vi "color.vi"(8 "error in":errorcluster, 11 "Stop (F) in":bool caption="Stop (F)") -> (0 "error out":errorcluster, 1 "blue":i32, 2 "red":i32, 3 "Refnum out":T1(plugin-control), 4 "yellow":i32, 5 "green":i32, 6 "Matches (Color Location 1) 2":T2(array[cluster]) {"Bounding Box"."y" format="%.2f"; "Bounding Box"."x" format="%.2f"; "Position"."y" format="%.2f"; "Position"."x" format="%.2f"; "Score" format="%.2f"; "Scale" format="%.2f"; "Angle" format="%.2f"}, 7 "black":i32)   [LabVIEW 2019]
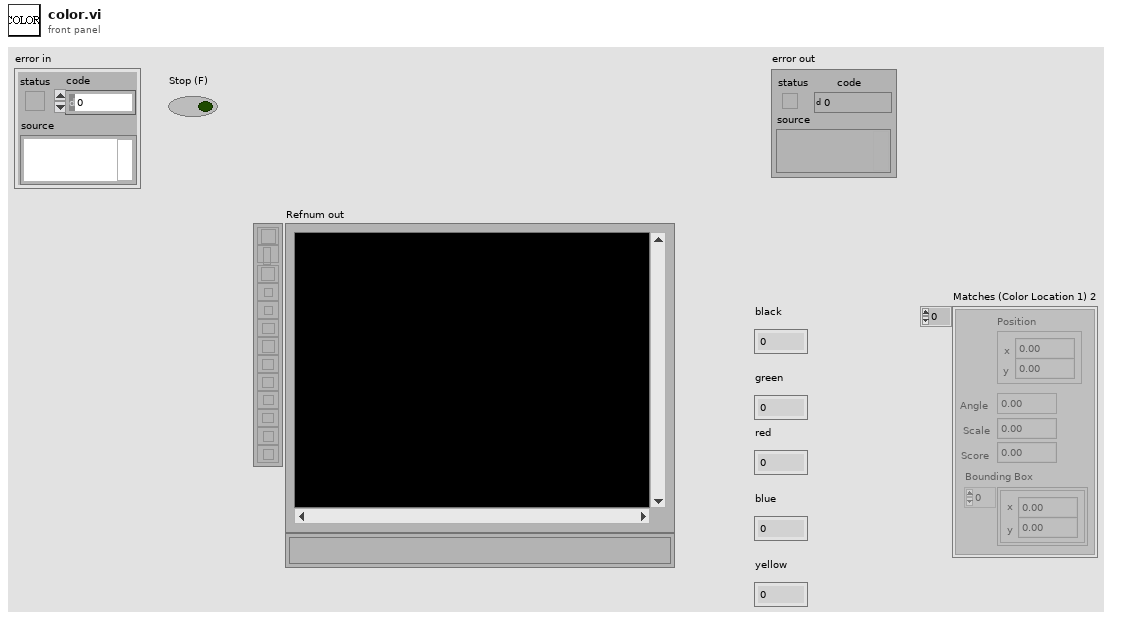
[diagram p1: front panel]
types:
  T1 = typedef "IMAQ Image.ctl" = refnum<image>
  T2 = cluster{"Position":cluster{"x":sgl, "y":sgl}, "Angle":sgl, "Scale":sgl, "Score":sgl, "Bounding Box":cluster{"x":sgl, "y":sgl}[]}[]
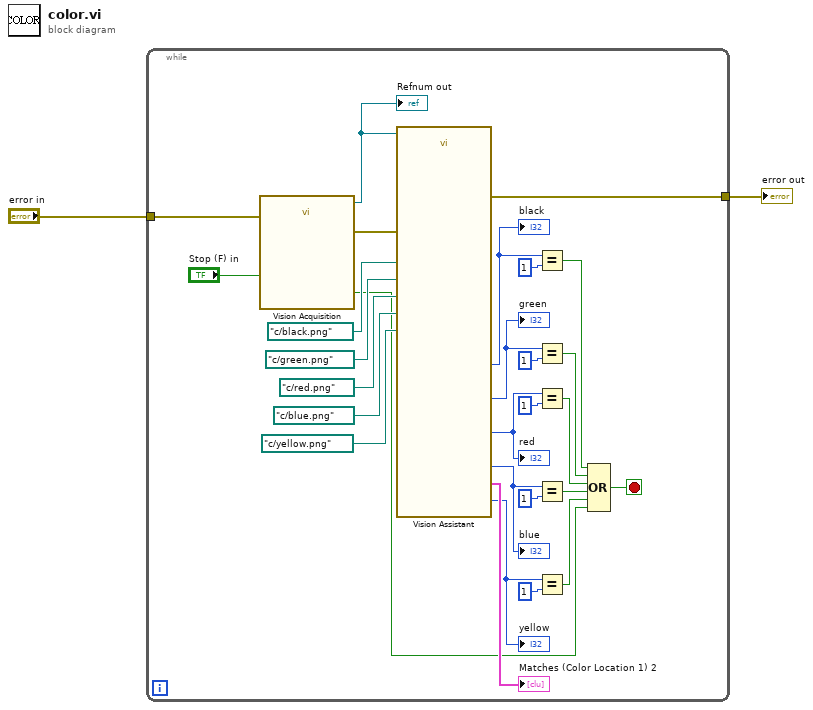
[diagram p0: block diagram]
diagram:
  n1 = while {
    tunnel: [w20] -> w2
    tunnel: "error in" -> [w3]
    stop <- w19 stop-if-true
    n2 = call "Vision Acquisition"("Stop (F)"="Stop (F) in", "error in"=w3) -> ("Image Out"=w23:T1, "Stopped"=w17:bool, "error out"=w21:errorcluster)  [unwired: 23 in]
    "Refnum out" <- w23
    n3 = call "Vision Assistant"("Image In"=w23, "File Path (Color Location 1)"=path "c:/yellow.png", "File Path (Color Location 2)"=path "c:/blue.png", "File Path (Color Location 3)"=path "c:/red.png", "File Path (Color Location 4)"=path "c:/green.png", "File Path (Color Location 5)"=path "c:/black.png", "error in"=w21) -> ("Number of Matches (Color Location 5)"=w7:i32, "Number of Matches (Color Location 4)"=w4:i32, "Matches (Color Location 1)"=→"Matches (Color Location 1) 2":T2, "Number of Matches (Color Location 1)"=w8:i32, "Number of Matches (Color Location 2)"=w5:i32, "Number of Matches (Color Location 3)"=w6:i32, "error out"=w20:errorcluster)  [unwired: 9 in, 5 out]
    "black" <- w7
    "green" <- w4
    "red" <- w6
    "yellow" <- w8
    "blue" <- w5
    n4 = Equal?(x=w7, y=1) -> (x = y?=w9:bool)
    n5 = Equal?(x=w4, y=1) -> (x = y?=w10:bool)
    n6 = Equal?(x=w6, y=1) -> (x = y?=w11:bool)
    n7 = Equal?(x=w5, y=1) -> (x = y?=w15:bool)
    n8 = Equal?(x=w8, y=1) -> (x = y?=w18:bool)
    n9 = Compound Arithmetic op=OR(w9, w10, w11, w15, w18, w17) -> (w19:bool)
  }
  "error out" <- w2
